vi "LinearSystemId_DiffDrv_ID_Pack_Model_Params.vi"(8 "Ka Angular":dbl, 9 "Kv Angular":dbl, 10 "Ka Linear":dbl, 11 "Kv Linear":dbl) -> (3 "DiffDrv_LinearSystem":T1)   [LabVIEW 2019, in "Trajectory_Library.lvlib"]
uses:
  TypeDef/LINEAR_SYSTEM.ctl
  <vilib>/Analysis/Matrix/Datatypes/RealMatrix.ctl
  LinearSystem_New.vi
  MatBuilder_Create.vi
  MatBuilder_Fill.vi
  MatrixHelper_Zero.vi
  DCMotor_GetCIM.vi
  DCMotor_GetAndymark9015.vi
  DCMotor_GetAndymarkRs775_125.vi
  DCMotor_GetBag.vi
  DCMotor_GetBanebotsRs550.vi
  DCMotor_GetBanebotsRs775.vi
  DCMotor_GetFalcon500.vi
  DCMotor_GetMiniCIM.vi
  DCMotor_GetNEO.vi
  DCMotor_GetNEO550.vi
  DCMotor_GetRomiBuiltIn.vi
  DCMotor_GetVex775Pro.vi
  DCMotor_GetAndymarkAM2235A.vi
  DCMotor_GetAndymarkAM3493.vi
  MatrixHelper_CoerceSize.vi
  DCMotor_New.vi
  Units_RotationsPerMinuteToRadiansPerSecond.vi
  Trajectory_Library.lvlib
  <vilib>/Analysis/Matrix/NI_Matrix.lvlib
panel:
  # "<States,States>"
  # "<States,Inputs>"
  # "<Outputs,States>"
  # "<Outputs,Inputs>"
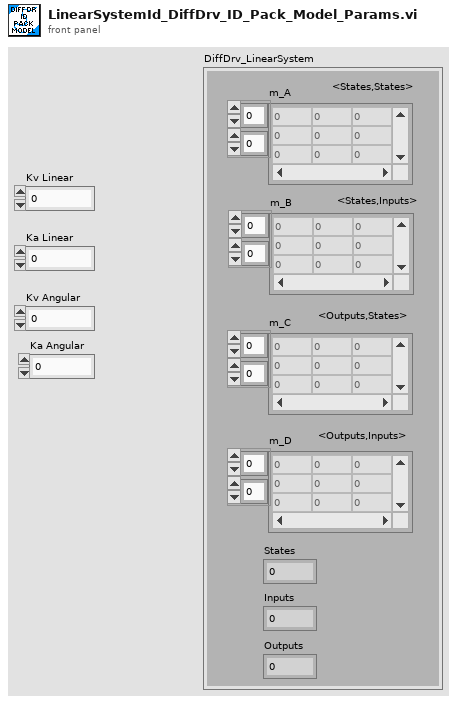
[diagram p1: front panel]
types:
  T1 = typedef "Trajectory_Library.lvlib/LINEAR_SYSTEM.ctl" = cluster{"m_A":T2, "m_B":T2, "m_C":T2, "m_D":T2, "States":i32, "Inputs":i32, "Outputs":i32}
  T2 = typedef "NI_Matrix.lvlib/RealMatrix.ctl" = dbl[][]
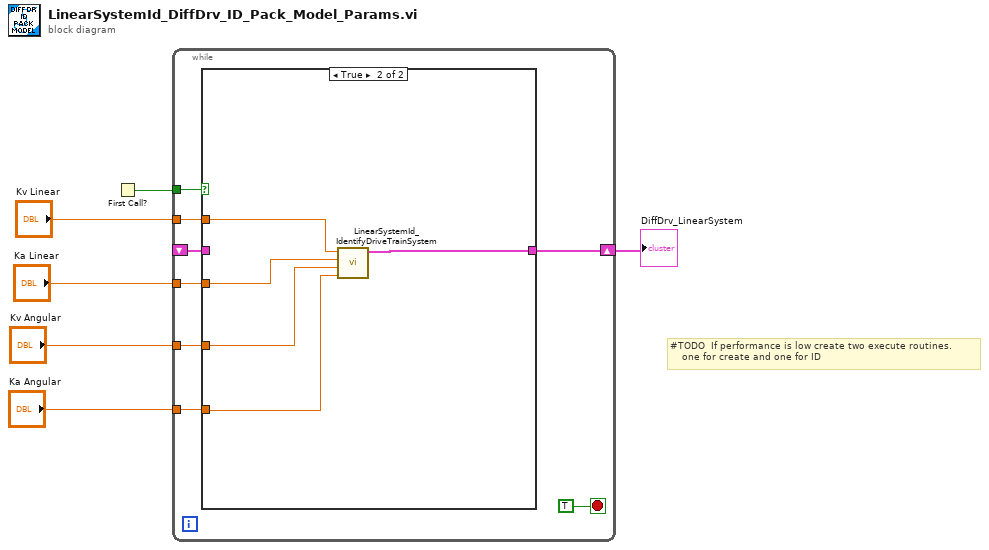
[diagram p0: block diagram]
diagram:
  # "#TODO  If performance is low create two execute routines.\n    one for create and one for ID"
  n1 = First Call?() -> (First Call?: T/F=w2:bool)
  n2 = while {
    tunnel: "Kv Linear" -> [w13]
    tunnel: "Ka Linear" -> [w12]
    tunnel: "Kv Angular" -> [w11]
    tunnel: "Ka Angular" -> [w10]
    shift-right: [w9] -> w1
    shift-left: _ -> [w7]
    tunnel: w2 -> [w8]
    stop <- TRUE stop-if-true
    n3 = case shown="True" w8 {
      tunnel: w13 -> [_ w20]
      tunnel: w12 -> [_ w19]
      tunnel: w11 -> [_ w18]
      tunnel: w10 -> [_ w17]
      tunnel: [w15 w16] -> w9
      tunnel: w7 -> [w15 _]
      frame False {
      }
      frame True {
        n4 = call "LinearSystemId_IdentifyDriveTrainSystem.vi"("kAAngular"=w17, "kVAngular"=w18, "kALinear"=w19, "kVLinear"=w20) -> ("Linearsystem"=w16:T1)  [unwired: 6 in, 1 out]
      }
    }
  }
  "DiffDrv_LinearSystem" <- w1
